vi "GV PreframegateDelayed.vi"() -> ()   [LabVIEW 2017]
panel:
  out "PreframegateDelayed":bool
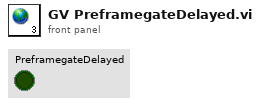
[diagram p1: front panel]
diagram:
